vi "Propagate Parent State.vi"(8 "error in (no error)":errorcluster, 10 "Target State in":refnum<class "State Machine Actor.lvclass">, 11 "State Machine Actor in":refnum<class "State Machine Actor.lvclass">) -> (0 "error out":errorcluster, 2 "Target State out":refnum<class "State Machine Actor.lvclass">, 3 "State Machine Actor out":refnum<class "State Machine Actor.lvclass">)   [LabVIEW 2024, in "State Machine Actor.lvlib" / "State Machine Actor.lvclass"]
doc: "Used to propagate the parent state for external transitions (that could be ocurring within a parent state)."
uses:
  State Machine Actor.lvclass
  State Machine Actor.lvclass/State Machine Actor.ctl
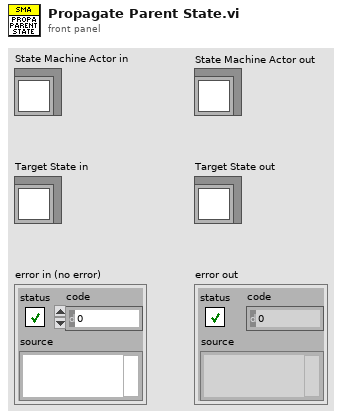
[diagram p1: front panel]
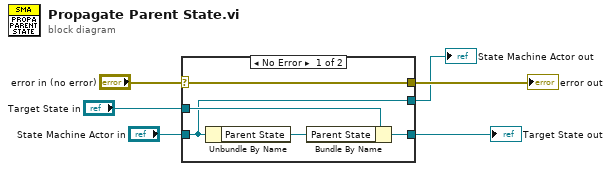
[diagram p0: block diagram]
diagram:
  n1 = case shown="No Error" "error in (no error)" {
    selector: "error in (no error)" -> [w11 w14]
    tunnel: [w11 w14] -> w5
    tunnel: [w8 w12] -> w3
    tunnel: "State Machine Actor in" -> [w7 w13]
    tunnel: "Target State in" -> [w9 w12]
    tunnel: [w7 w13] -> w1
    frame No Error {
      # "used to propagate the parent state for external transitions"
      n2 = Unbundle By Name(w7) -> ("Parent State"=w10:refnum<class "_State Machine Actor.lvclass">)
      n3 = Bundle By Name(cluster=w9, "Parent State"=w10) -> (w8:refnum<class "State Machine Actor.lvclass">)
    }
    frame Error {
    }
  }
  "error out" <- w5
  "Target State out" <- w3
  "State Machine Actor out" <- w1
